vi "ep_Detect Voltage Events.vi"(0 "event limits":T5(array[cluster]), 1 "restart (F)":bool, 5 "voltage RMS (1/2) (1 cycle)":T4(array[cluster]), 7 "polyphase only? (F)":bool, 11 "error in (no error)":errorcluster) -> (4 "voltage events":T3(array[cluster]), 10 "voltage flags":bool[](array[boolean]), 15 "error out":errorcluster)   [LabVIEW 2014, in "NI_EP_Power Quality.lvlib"]
uses:
  <vilib>/addons/Electrical Power/PQ/NI_EP_Power Quality.lvlib
  <vilib>/addons/Electrical Power/PQ/Common/Controls/ep_Phase.ctl
  <vilib>/addons/Electrical Power/PQ/Common/Controls/ep_Event Type.ctl
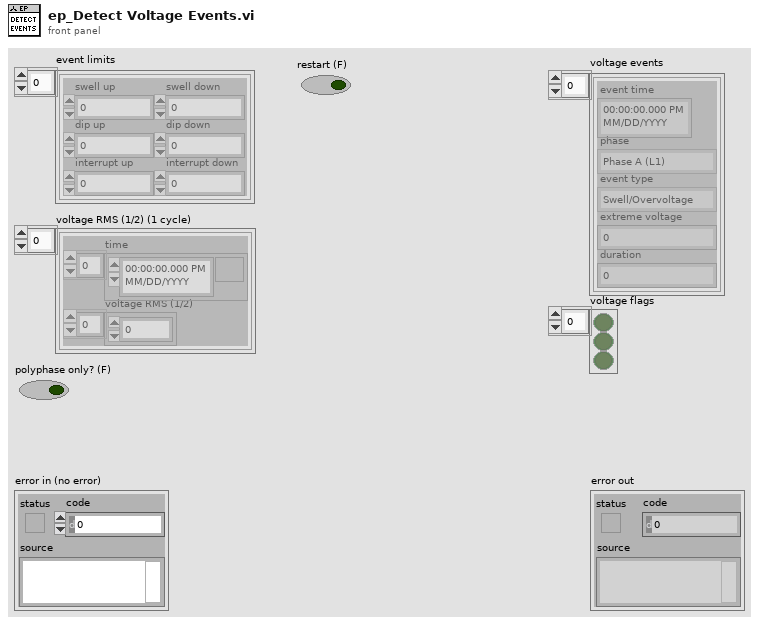
[diagram p1: front panel]
types:
  T1 = typedef "NI_EP_Power Quality.lvlib/ep_Phase.ctl" = enum16{"Phase A (L1)", "Phase B (L2)", "Phase C (L3)", "Phase N", "~3 Phases"}
  T2 = typedef "NI_EP_Power Quality.lvlib/ep_Event Type.ctl" = enum16{"Swell/Overvoltage", "Dip/Undervoltage", "Interruption"}
  T3 = cluster{"event time":timestamp, "phase":T1, "event type":T2, "extreme voltage":dbl, "duration":dbl}[]
  T4 = cluster{"time":timestamp[], "voltage RMS (1/2)":dbl[]}[]
  T5 = cluster{"swell up":dbl, "swell down":dbl, "dip up":dbl, "dip down":dbl, "interrupt up":dbl, "interrupt down":dbl}[]
  T6 = cluster{"event time":timestamp, "voltage RMS":dbl, "phase":T1}[]
  T7 = cluster{"event time":timestamp, "voltage RMS":dbl, "phase":T1}
  T8 = cluster{"swell up":dbl, "swell down":dbl, "dip up":dbl, "dip down":dbl, "interrupt up":dbl, "interrupt down":dbl}
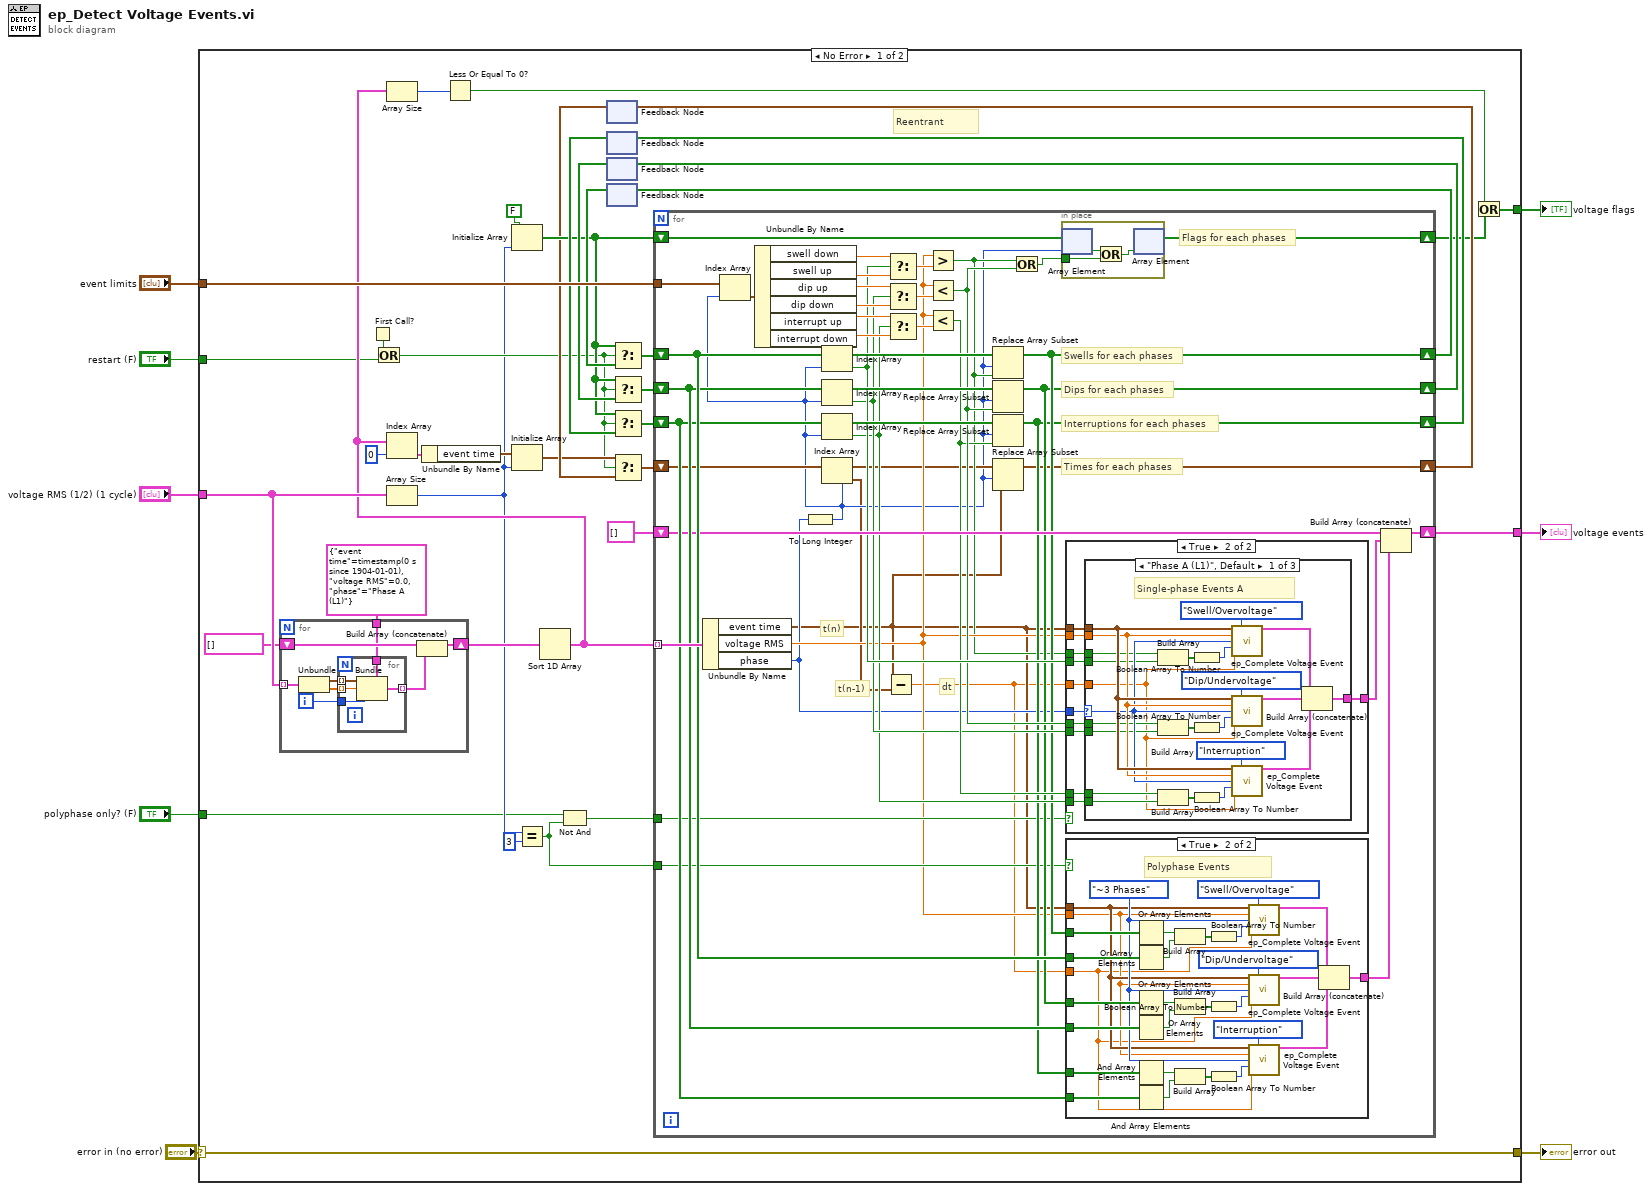
[diagram p0: block diagram]
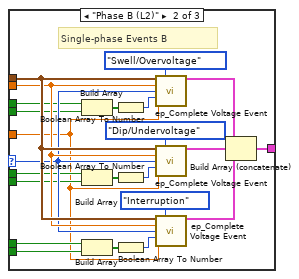
[diagram p3: hidden frame]
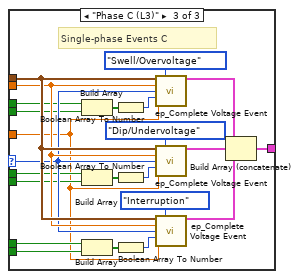
[diagram p4: hidden frame]
diagram:
  n1 = case shown="No Error" "error in (no error)" {
    selector: "error in (no error)" -> [w14 w214]
    tunnel: "event limits" -> [w46 _]
    tunnel: "voltage RMS (1/2) (1 cycle)" -> [w42 _]
    tunnel: [w37 _] -> w6
    tunnel: [w28 _] -> w5
    tunnel: "restart (F)" -> [w26 _]
    tunnel: "polyphase only? (F)" -> [w10 _]
    tunnel: [w14 w214] -> w1
    frame No Error {
      # "Reentrant"
      n2 = for {
        tunnel: w42 -> [w208] mode=indexing
        shift-right: [w203] -> w47
        shift-left: T6 [] -> [w202]
        tunnel: T7 {"event time"=timestamp(0 s since 1904-01-01), "voltage RMS"=0.0, "phase"=enum."Phase A (L1)"} ("voltage event") -> [w201]
        i -> [w205]
        n3 = Unbundle(w208) -> ("time"=w207:timestamp[], "voltage RMS (1/2)"=w206:dbl[])
        n4 = for {
          tunnel: w207 -> [w213] mode=indexing
          tunnel: w206 -> [w212] mode=indexing
          tunnel: w205 -> [w211]
          tunnel: [w210] -> w204 mode=indexing
          tunnel: w201 -> [w209]
          n5 = Bundle(cluster=w209, "event time"=w213, "voltage RMS"=w212, "phase"=w211) -> (w210:T7)
        }
        n6 = Build Array (concatenate)(w202, w204) -> (w203:T6)
      }
      n7 = First Call?() -> (First Call?: T/F=w27:bool)
      n8 = Or(x=w27, y=w26) -> (x .or. y?=w15:bool)
      n9 = Array Size(array=w42) -> (size(s)=w13:i32)
      n10 = Initialize Array(FALSE, w13) -> (w19:bool[])
      n11 = Equal?(x=w13, y=3) -> (x = y?=w9:bool)
      n12 = Sort 1D Array(array=w47) -> (sorted array=w32:T6)
      n13 = Array Size(array=w32) -> (size(s)=w31:i32)
      n14 = Index Array(array=w32, index=0) -> (element=w34:T7)
      n15 = Unbundle By Name(w34) -> ("event time"=w35:timestamp)
      n16 = Less Or Equal To 0?(x=w31) -> (x <= 0?=w30:bool)
      n17 = Initialize Array(w35, w13) -> (w16:timestamp[])
      n18 = Not And(1:w9, 2:w10) -> (0:w11:bool)
      n19 = feedback #1() -> (w18:timestamp[])  [unwired: 1 in]
      n20 = feedback #2() -> (w23:bool[])  [unwired: 1 in]
      n21 = feedback #3() -> (w22:bool[])  [unwired: 1 in]
      n22 = feedback #4() -> (w25:bool[])  [unwired: 1 in]
      n23 = Select(t=w19, s=w15, f=w25) -> (s? t:f=w24:bool[])
      n24 = Select(t=w19, s=w15, f=w22) -> (s? t:f=w21:bool[])
      n25 = Select(t=w19, s=w15, f=w23) -> (s? t:f=w20:bool[])
      n26 = Select(t=w16, s=w15, f=w18) -> (s? t:f=w17:timestamp[])
      n27 = for {
        tunnel: w32 -> [w88] mode=indexing
        tunnel: w46 -> [w87]
        shift-right: [w63] -> w44
        shift-left: w24 -> [w73]
        shift-right: [w62] -> w41
        shift-left: w21 -> [w72]
        shift-right: [w61] -> w40
        shift-left: w20 -> [w71]
        shift-right: [w74] -> w29
        shift-left: w19 -> [w76]
        shift-right: [w69] -> w37
        shift-left: T3 [] ("voltage events") -> [w70]
        tunnel: w11 -> [w58]
        tunnel: w9 -> [w57]
        shift-right: [w54] -> w36
        shift-left: w17 -> [w53]
        # "dt"
        # "t(n-1)"
        # "t(n)"
        # "Times for each phases"
        # "Flags for each phases"
        # "Interruptions for each phases"
        # "Dips for each phases"
        # "Swells for each phases"
        n28 = Unbundle By Name(w88) -> ("event time"=w49:timestamp, "voltage RMS"=w56:dbl, "phase"=w52:T1)
        n29 = To Long Integer(number=w52) -> (32bit integer=w51:i32)
        n30 = Index Array(array=w87, index=w51) -> (element=w83:T8)
        n31 = Unbundle By Name(w83) -> ("swell down"=w86:dbl, "swell up"=w85:dbl, "dip up"=w77:dbl, "dip down"=w78:dbl, "interrupt up"=w79:dbl, "interrupt down"=w80:dbl)
        n32 = Index Array(array=w73, index=w51) -> (element=w68:bool)
        n33 = Index Array(array=w72, index=w51) -> (element=w65:bool)
        n34 = Index Array(array=w71, index=w51) -> (element=w64:bool)
        n35 = Index Array(array=w53, index=w51) -> (element=w50:timestamp)
        n36 = Subtract(x=w49, y=w50) -> (x-y=w48:dbl)
        n37 = Select(t=w86, s=w68, f=w85) -> (s? t:f=w84:dbl)
        n38 = Select(t=w77, s=w65, f=w78) -> (s? t:f=w82:dbl)
        n39 = Select(t=w79, s=w64, f=w80) -> (s? t:f=w81:dbl)
        n40 = Greater?(x=w56, y=w84) -> (0:w55:bool)
        n41 = Less?(x=w56, y=w82) -> (x < y?=w67:bool)
        n42 = Less?(x=w56, y=w81) -> (x < y?=w66:bool)
        n43 = Replace Array Subset(array=w73, new element=w55, index=w51) -> (w63:bool[])
        n44 = Replace Array Subset(array=w72, new element=w67, index=w51) -> (w62:bool[])
        n45 = Replace Array Subset(array=w71, new element=w66, index=w51) -> (w61:bool[])
        n46 = Replace Array Subset(array=w53, new element=w49, index=w51) -> (w54:timestamp[])
        n47 = Or(x=w55, y=w67) -> (x .or. y?=w75:bool)
        n48 = in-place {
          in-place-border: w75 -> [w198]
          n49 = in-place-array #5(w76, w51) -> (w200:bool)
          n50 = Or(x=w200, y=w198) -> (x .or. y?=w199:bool)
          n51 = in-place-array #5(w199) -> (w74:bool[])  [unwired: 1 out]
        }
        n52 = case shown="True" w58 {
          tunnel: w49 -> [_ w99]
          tunnel: w56 -> [_ w98]
          tunnel: w52 -> [_ w97]
          tunnel: w55 -> [_ w96]
          tunnel: w68 -> [_ w95]
          tunnel: w67 -> [_ w94]
          tunnel: w66 -> [_ w93]
          tunnel: w65 -> [_ w92]
          tunnel: w64 -> [_ w91]
          tunnel: [_ w90] -> w60
          tunnel: w48 -> [_ w89]
          frame False {
          }
          frame True {
            n53 = case shown="\"Phase A (L1)\", Default" w97 {
              selector: w97 -> [w107 w130 w153]
              tunnel: w99 -> [w113 w136 w159]
              tunnel: w98 -> [w112 w135 w158]
              tunnel: [w108 w131 w154] -> w90
              tunnel: w96 -> [w106 w129 w152]
              tunnel: w95 -> [w105 w128 w151]
              tunnel: w94 -> [w104 w127 w150]
              tunnel: w93 -> [w103 w126 w149]
              tunnel: w92 -> [w102 w125 w148]
              tunnel: w91 -> [w101 w124 w147]
              tunnel: w89 -> [w100 w123 w146]
              frame "Phase A (L1)", Default {
                # "Single-phase Events A"
                n54 = Build Array(w106, w105) -> (w120:bool[])
                n55 = Build Array(w104, w102) -> (w119:bool[])
                n56 = Build Array(w103, w101) -> (w114:bool[])
                n57 = Boolean Array To Number(Boolean array=w120) -> (number=w121:u32)
                n58 = Boolean Array To Number(Boolean array=w119) -> (number=w118:u32)
                n59 = Boolean Array To Number(Boolean array=w114) -> (number=w115:u32)
                n60 = call <vilib>:"ep_Complete Voltage Event.vi"("time"=w113, "event type"=ep_Event_Type."Swell/Overvoltage", "voltage RMS"=w112, "phase"=w107, "event state"=w121, "dt"=w100) -> ("voltage events"=w111:T3)  [unwired: 9 in]
                n61 = call <vilib>:"ep_Complete Voltage Event.vi"("time"=w113, "event type"=ep_Event_Type."Dip/Undervoltage", "voltage RMS"=w112, "phase"=w107, "event state"=w118, "dt"=w100) -> ("voltage events"=w109:T3)  [unwired: 9 in]
                n62 = call <vilib>:"ep_Complete Voltage Event.vi"("time"=w113, "event type"=ep_Event_Type."Interruption", "voltage RMS"=w112, "phase"=w107, "event state"=w115, "dt"=w100) -> ("voltage events"=w110:T3)  [unwired: 9 in]
                n63 = Build Array (concatenate)(w111, w109, w110) -> (w108:T3)
              }
              frame "Phase B (L2)" {
                # "Single-phase Events B"
                n64 = Build Array(w129, w128) -> (w143:bool[])
                n65 = Build Array(w127, w125) -> (w142:bool[])
                n66 = Build Array(w126, w124) -> (w137:bool[])
                n67 = Boolean Array To Number(Boolean array=w143) -> (number=w144:u32)
                n68 = Boolean Array To Number(Boolean array=w142) -> (number=w141:u32)
                n69 = Boolean Array To Number(Boolean array=w137) -> (number=w138:u32)
                n70 = call <vilib>:"ep_Complete Voltage Event.vi"("time"=w136, "event type"=ep_Event_Type."Swell/Overvoltage", "voltage RMS"=w135, "phase"=w130, "event state"=w144, "dt"=w123) -> ("voltage events"=w134:T3)  [unwired: 9 in]
                n71 = call <vilib>:"ep_Complete Voltage Event.vi"("time"=w136, "event type"=ep_Event_Type."Dip/Undervoltage", "voltage RMS"=w135, "phase"=w130, "event state"=w141, "dt"=w123) -> ("voltage events"=w132:T3)  [unwired: 9 in]
                n72 = call <vilib>:"ep_Complete Voltage Event.vi"("time"=w136, "event type"=ep_Event_Type."Interruption", "voltage RMS"=w135, "phase"=w130, "event state"=w138, "dt"=w123) -> ("voltage events"=w133:T3)  [unwired: 9 in]
                n73 = Build Array (concatenate)(w134, w132, w133) -> (w131:T3)
              }
              frame "Phase C (L3)" {
                # "Single-phase Events C"
                n74 = Build Array(w152, w151) -> (w166:bool[])
                n75 = Build Array(w150, w148) -> (w165:bool[])
                n76 = Build Array(w149, w147) -> (w160:bool[])
                n77 = Boolean Array To Number(Boolean array=w166) -> (number=w167:u32)
                n78 = Boolean Array To Number(Boolean array=w165) -> (number=w164:u32)
                n79 = Boolean Array To Number(Boolean array=w160) -> (number=w161:u32)
                n80 = call <vilib>:"ep_Complete Voltage Event.vi"("time"=w159, "event type"=ep_Event_Type."Swell/Overvoltage", "voltage RMS"=w158, "phase"=w153, "event state"=w167, "dt"=w146) -> ("voltage events"=w157:T3)  [unwired: 9 in]
                n81 = call <vilib>:"ep_Complete Voltage Event.vi"("time"=w159, "event type"=ep_Event_Type."Dip/Undervoltage", "voltage RMS"=w158, "phase"=w153, "event state"=w164, "dt"=w146) -> ("voltage events"=w155:T3)  [unwired: 9 in]
                n82 = call <vilib>:"ep_Complete Voltage Event.vi"("time"=w159, "event type"=ep_Event_Type."Interruption", "voltage RMS"=w158, "phase"=w153, "event state"=w161, "dt"=w146) -> ("voltage events"=w156:T3)  [unwired: 9 in]
                n83 = Build Array (concatenate)(w157, w155, w156) -> (w154:T3)
              }
            }
          }
        }
        n84 = case shown="True" w57 {
          tunnel: w63 -> [_ w187]
          tunnel: w73 -> [_ w186]
          tunnel: w62 -> [_ w185]
          tunnel: w72 -> [_ w184]
          tunnel: w61 -> [_ w178]
          tunnel: w71 -> [_ w177]
          tunnel: w49 -> [_ w175]
          tunnel: w56 -> [_ w174]
          tunnel: [_ w170] -> w59
          tunnel: w48 -> [_ w169]
          frame False {
          }
          frame True {
            w176 = ep_Phase."~3 Phases" ("phase")
            # "Polyphase Events"
            n85 = Or Array Elements(Boolean array=w187) -> (logical OR=w194:bool)
            n86 = Or Array Elements(Boolean array=w186) -> (logical OR=w193:bool)
            n87 = Or Array Elements(Boolean array=w185) -> (logical OR=w191:bool)
            n88 = Or Array Elements(Boolean array=w184) -> (logical OR=w192:bool)
            n89 = And Array Elements(Boolean array=w178) -> (logical AND=w180:bool)
            n90 = And Array Elements(Boolean array=w177) -> (logical AND=w179:bool)
            n91 = Build Array(w194, w193) -> (w195:bool[])
            n92 = Build Array(w191, w192) -> (w190:bool[])
            n93 = Build Array(w180, w179) -> (w181:bool[])
            n94 = Boolean Array To Number(Boolean array=w195) -> (number=w196:u32)
            n95 = Boolean Array To Number(Boolean array=w190) -> (number=w189:u32)
            n96 = Boolean Array To Number(Boolean array=w181) -> (number=w182:u32)
            n97 = call <vilib>:"ep_Complete Voltage Event.vi"("time"=w175, "event type"=ep_Event_Type."Swell/Overvoltage", "voltage RMS"=w174, "phase"=w176, "event state"=w196, "dt"=w169) -> ("voltage events"=w173:T3)  [unwired: 9 in]
            n98 = call <vilib>:"ep_Complete Voltage Event.vi"("time"=w175, "event type"=ep_Event_Type."Dip/Undervoltage", "voltage RMS"=w174, "phase"=w176, "event state"=w189, "dt"=w169) -> ("voltage events"=w171:T3)  [unwired: 9 in]
            n99 = call <vilib>:"ep_Complete Voltage Event.vi"("time"=w175, "event type"=ep_Event_Type."Interruption", "voltage RMS"=w174, "phase"=w176, "event state"=w182, "dt"=w169) -> ("voltage events"=w172:T3)  [unwired: 9 in]
            n100 = Build Array (concatenate)(w173, w171, w172) -> (w170:T3)
          }
        }
        n101 = Build Array (concatenate)(w70, w60, w59) -> (w69:T3)
      }
      n102 = feedback-in #1(w36) -> ()
      n103 = feedback-in #2(w40) -> ()
      n104 = feedback-in #3(w41) -> ()
      n105 = feedback-in #4(w44) -> ()
      n106 = Or(x=w30, y=w29) -> (x .or. y?=w28:bool[])
    }
    frame Error {
    }
  }
  "voltage flags" <- w5
  "voltage events" <- w6
  "error out" <- w1
